vi "FTW-Message-Decompose.vi"(0 "Multipart Message":string[](array[string])) -> (2 "Sender Identity":string, 3 "Message Header":string, 4 "Message Body":string)   [LabVIEW 2013, in "FTW-Message.lvclass"]
uses:
  FTW-Message.lvclass
panel:
  # "Inputs"
  # "Outputs"
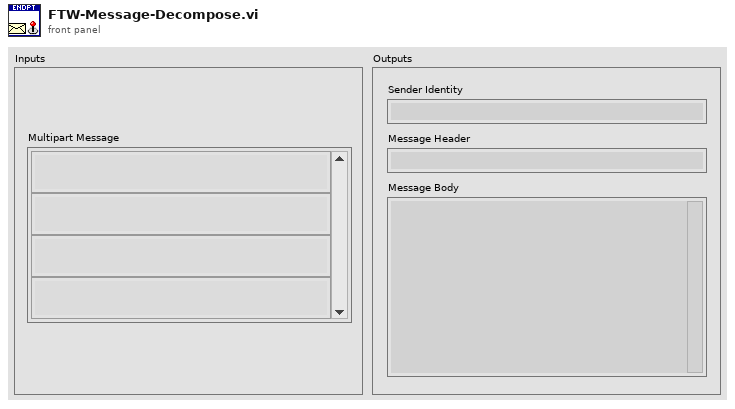
[diagram p1: front panel]
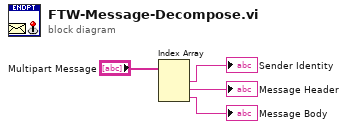
[diagram p0: block diagram]
diagram:
  n1 = Index Array(array="Multipart Message") -> (element #1=→"Sender Identity":string, element #2=→"Message Header":string, element #3=→"Message Body":string)  [unwired: 3 in]
